vi "CODMn手动控制框.vi"(8 "Error in":errorcluster) -> ()   [LabVIEW 2016, in "斯坦道CODMn.lvlib"]
uses:
  <vilib>/Plasmionique/MB Master/MB Master.lvlib
panel:
  out "退出 2":bool
  in  "采水泵排":bool
  in  "采水泵进":bool
  in  "草酸钠":bool
  in  "高锰酸钾":bool
  in  "高锰酸钾滴定（10uL每滴）":bool
  in  "草酸钠泵排":bool
  in  "草酸钠泵进":bool
  in  "草酸钠泵复位":bool
  in  "高锰酸钾泵排":bool
  in  "高锰酸钾泵进":bool
  in  "高锰酸钾泵复位":bool
  in  "风扇":bool
  in  "排液":bool
  in  "搅拌":bool
  in  "加热":bool
  in  "硫酸":bool
  in  "加标回收样":bool
  in  "零点核查样":bool
  in  "标液":bool
  in  "纯水":bool
  in  "退出":bool
  in  "水样":bool
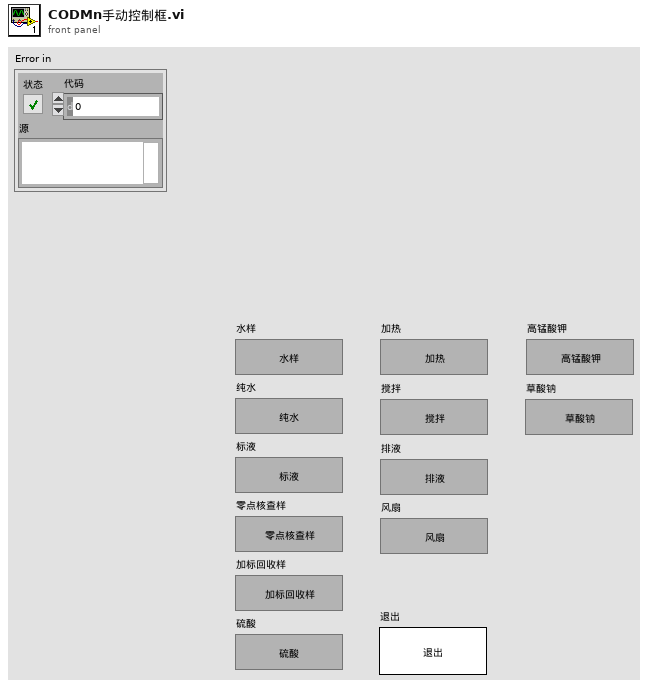
[diagram p1: front panel]
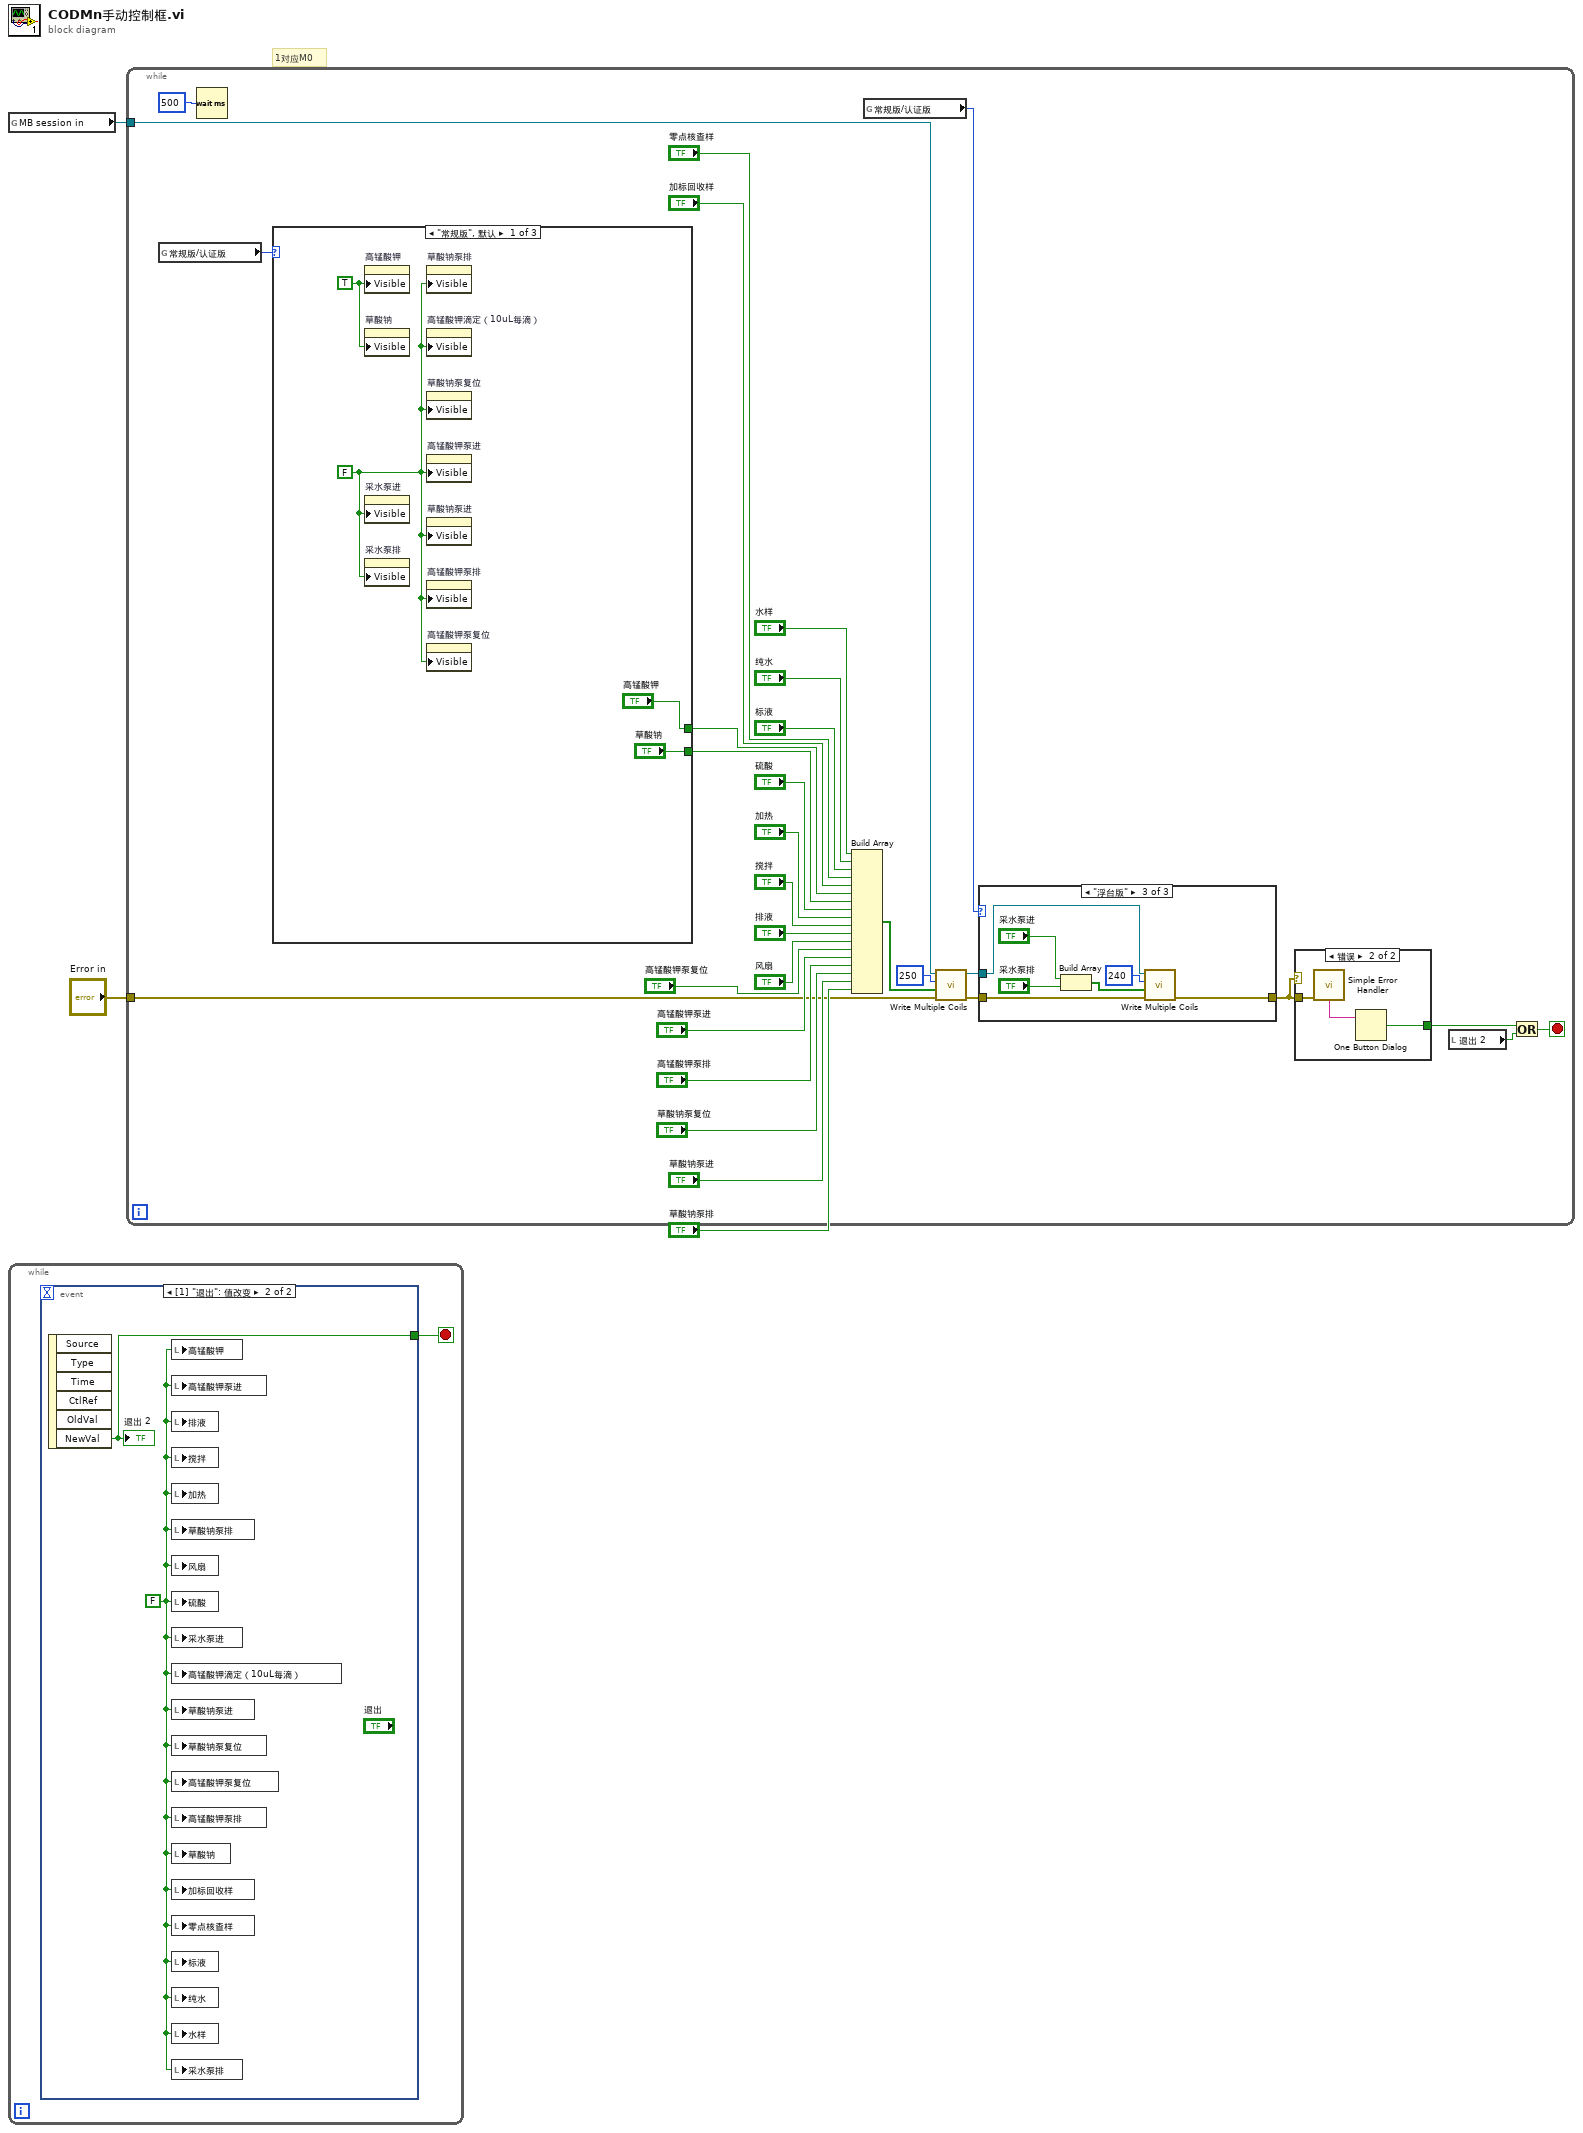
[diagram p0: block diagram]
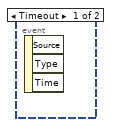
[diagram p2: hidden frame]
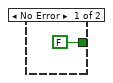
[diagram p3: hidden frame]
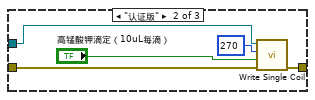
[diagram p5: hidden frame]
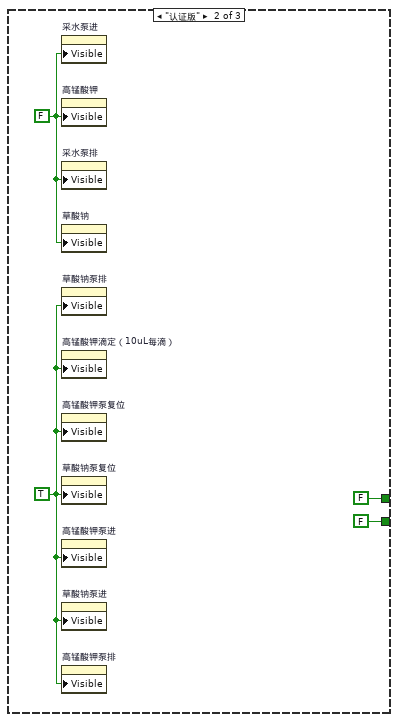
[diagram p6: hidden frame]
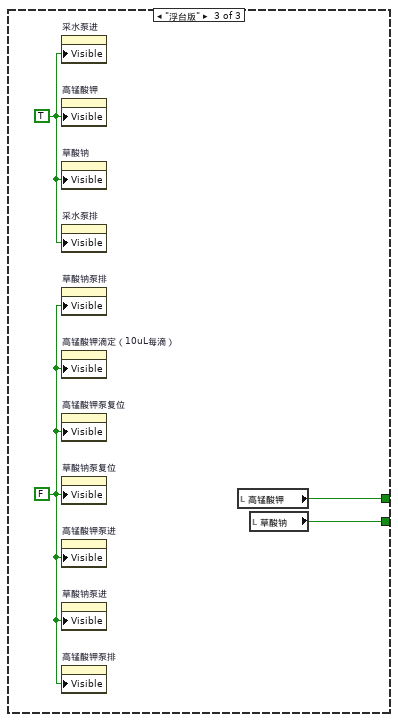
[diagram p7: hidden frame]
diagram:
  # "1对应M0"
  n1 = global read "COD浓度全局变量.vi" "MB session in"() -> (w1:refnum<class "MB_Master.lvclass">)
  n2 = while {
    stop <- w3 stop-if-true
    n3 = event shown="[1] \"退出\": 值改变" {
      selector: _ -> [_ _]
      dyn-events: _ -> [_ _]
      timeout: _ -> [_ _]
      tunnel: [_ w5] -> w3
      event Timeout {
        n4 = event-data() -> ()  [unwired: 1 in, 3 out]
      }
      event "退出": Value Change {
        w4 = FALSE ("草酸钠")
        n5 = event-data() -> ("NewVal"=w5:bool)  [unwired: 1 in, 5 out]
        "退出 2" <- w5
        n6 = local write "高锰酸钾"(w4) -> ()
        n7 = local write "高锰酸钾泵进"(w4) -> ()
        n8 = local write "排液"(w4) -> ()
        n9 = local write "搅拌"(w4) -> ()
        n10 = local write "加热"(w4) -> ()
        n11 = local write "草酸钠泵排"(w4) -> ()
        n12 = local write "风扇"(w4) -> ()
        n13 = local write "硫酸"(w4) -> ()
        n14 = local write "采水泵进"(w4) -> ()
        n15 = local write "高锰酸钾滴定（10uL每滴）"(w4) -> ()
        n16 = local write "草酸钠泵进"(w4) -> ()
        n17 = local write "草酸钠泵复位"(w4) -> ()
        n18 = local write "高锰酸钾泵复位"(w4) -> ()
        n19 = local write "高锰酸钾泵排"(w4) -> ()
        n20 = local write "草酸钠"(w4) -> ()
        n21 = local write "加标回收样"(w4) -> ()
        n22 = local write "零点核查样"(w4) -> ()
        n23 = local write "标液"(w4) -> ()
        n24 = local write "纯水"(w4) -> ()
        n25 = local write "水样"(w4) -> ()
        n26 = local write "采水泵排"(w4) -> ()
      }
    }
  }
  n27 = while {
    tunnel: "Error in" -> [w17]
    tunnel: w1 -> [w12]
    stop <- w9 stop-if-true
    n28 = global read "CODMn断电保存全局变量.vi" "常规版/认证版"() -> (w8:enum16{"常规版", "认证版", "浮台版"})
    n29 = Wait (ms)(milliseconds to wait=u32 500 ("等待时间（毫秒）")) -> ()  [unwired: 1 out]
    n30 = case shown="\"常规版\", 默认" w8 {
      tunnel: ["高锰酸钾" FALSE ("元素") w64] -> w14
      tunnel: ["草酸钠" FALSE ("元素") w63] -> w13
      frame "常规版", Default {
        w54 = FALSE ("可见")
        w57 = TRUE ("可见")
        n31 = property on="高锰酸钾" class="Bool (严格)"("Visible"=w57) -> ()  [unwired: 2 in, 2 out]
        n32 = property on="草酸钠" class="Bool (严格)"("Visible"=w57) -> ()  [unwired: 2 in, 2 out]
        n33 = property on="采水泵进" class="Bool (严格)"("Visible"=w54) -> ()  [unwired: 2 in, 2 out]
        n34 = property on="采水泵排" class="Bool (严格)"("Visible"=w54) -> ()  [unwired: 2 in, 2 out]
        n35 = property on="草酸钠泵排" class="Bool (严格)"("Visible"=w54) -> ()  [unwired: 2 in, 2 out]
        n36 = property on="高锰酸钾滴定（10uL每滴）" class="Bool (严格)"("Visible"=w54) -> ()  [unwired: 2 in, 2 out]
        n37 = property on="草酸钠泵复位" class="Bool (严格)"("Visible"=w54) -> ()  [unwired: 2 in, 2 out]
        n38 = property on="高锰酸钾泵进" class="Bool (严格)"("Visible"=w54) -> ()  [unwired: 2 in, 2 out]
        n39 = property on="草酸钠泵进" class="Bool (严格)"("Visible"=w54) -> ()  [unwired: 2 in, 2 out]
        n40 = property on="高锰酸钾泵排" class="Bool (严格)"("Visible"=w54) -> ()  [unwired: 2 in, 2 out]
        n41 = property on="高锰酸钾泵复位" class="Bool (严格)"("Visible"=w54) -> ()  [unwired: 2 in, 2 out]
      }
      frame "认证版" {
        w61 = TRUE ("可见")
        w58 = FALSE ("可见")
        n42 = property on="采水泵进" class="Bool (严格)"("Visible"=w58) -> ()  [unwired: 2 in, 2 out]
        n43 = property on="高锰酸钾" class="Bool (严格)"("Visible"=w58) -> ()  [unwired: 2 in, 2 out]
        n44 = property on="采水泵排" class="Bool (严格)"("Visible"=w58) -> ()  [unwired: 2 in, 2 out]
        n45 = property on="草酸钠" class="Bool (严格)"("Visible"=w58) -> ()  [unwired: 2 in, 2 out]
        n46 = property on="草酸钠泵排" class="Bool (严格)"("Visible"=w61) -> ()  [unwired: 2 in, 2 out]
        n47 = property on="高锰酸钾滴定（10uL每滴）" class="Bool (严格)"("Visible"=w61) -> ()  [unwired: 2 in, 2 out]
        n48 = property on="高锰酸钾泵复位" class="Bool (严格)"("Visible"=w61) -> ()  [unwired: 2 in, 2 out]
        n49 = property on="草酸钠泵复位" class="Bool (严格)"("Visible"=w61) -> ()  [unwired: 2 in, 2 out]
        n50 = property on="高锰酸钾泵进" class="Bool (严格)"("Visible"=w61) -> ()  [unwired: 2 in, 2 out]
        n51 = property on="草酸钠泵进" class="Bool (严格)"("Visible"=w61) -> ()  [unwired: 2 in, 2 out]
        n52 = property on="高锰酸钾泵排" class="Bool (严格)"("Visible"=w61) -> ()  [unwired: 2 in, 2 out]
      }
      frame "浮台版" {
        w65 = FALSE ("可见")
        w62 = TRUE ("可见")
        n53 = property on="采水泵进" class="Bool (严格)"("Visible"=w62) -> ()  [unwired: 2 in, 2 out]
        n54 = property on="高锰酸钾" class="Bool (严格)"("Visible"=w62) -> ()  [unwired: 2 in, 2 out]
        n55 = property on="草酸钠" class="Bool (严格)"("Visible"=w62) -> ()  [unwired: 2 in, 2 out]
        n56 = property on="采水泵排" class="Bool (严格)"("Visible"=w62) -> ()  [unwired: 2 in, 2 out]
        n57 = property on="草酸钠泵排" class="Bool (严格)"("Visible"=w65) -> ()  [unwired: 2 in, 2 out]
        n58 = property on="高锰酸钾滴定（10uL每滴）" class="Bool (严格)"("Visible"=w65) -> ()  [unwired: 2 in, 2 out]
        n59 = property on="高锰酸钾泵复位" class="Bool (严格)"("Visible"=w65) -> ()  [unwired: 2 in, 2 out]
        n60 = property on="草酸钠泵复位" class="Bool (严格)"("Visible"=w65) -> ()  [unwired: 2 in, 2 out]
        n61 = property on="高锰酸钾泵进" class="Bool (严格)"("Visible"=w65) -> ()  [unwired: 2 in, 2 out]
        n62 = property on="草酸钠泵进" class="Bool (严格)"("Visible"=w65) -> ()  [unwired: 2 in, 2 out]
        n63 = property on="高锰酸钾泵排" class="Bool (严格)"("Visible"=w65) -> ()  [unwired: 2 in, 2 out]
        n64 = local read "高锰酸钾"() -> (w64:bool)
        n65 = local read "草酸钠"() -> (w63:bool)
      }
    }
    n66 = Build Array("水样", "纯水", "标液", "零点核查样", "加标回收样", w14, w13, "硫酸", "加热", "搅拌", "排液", "风扇", "高锰酸钾泵复位", "高锰酸钾泵进", "高锰酸钾泵排", "草酸钠泵复位", "草酸钠泵进", "草酸钠泵排") -> (w34:bool[])
    n67 = global read "CODMn断电保存全局变量.vi" "常规版/认证版"() -> (w7:enum16{"常规版", "认证版", "浮台版"})
    n68 = call <vilib>:"Write Multiple Coils.vi"("error in (no error)"=w17, "values"=w34, "starting address"=u16 250, "MB session in"=w12) -> ("error out"=w15:errorcluster, "MB session out"=w16:refnum<class "MB_Master.lvclass">)  [unwired: 6 in]
    n69 = case shown="\"浮台版\"" w7 {
      tunnel: w16 -> [_ w46 w53]
      tunnel: w15 -> [w41 w45 w52]
      tunnel: [w41 w42 w47] -> w11
      frame "常规版", Default {
      }
      frame "认证版" {
        n70 = call <vilib>:"Write Single Coil.vi"("error in (no error)"=w45, "value"="高锰酸钾滴定（10uL每滴）", "address"=u16 270 ("starting address"), "MB session in"=w46) -> ("error out"=w42:errorcluster)  [unwired: 6 in, 1 out]
      }
      frame "浮台版" {
        n71 = Build Array("采水泵进", "采水泵排") -> (w48:bool[])
        n72 = call <vilib>:"Write Multiple Coils.vi"("error in (no error)"=w52, "values"=w48, "starting address"=u16 240, "MB session in"=w53) -> ("error out"=w47:errorcluster)  [unwired: 6 in, 1 out]
      }
    }
    n73 = case shown="错误" w11 {
      tunnel: w11 -> [_ w40]
      tunnel: [FALSE ("true") w38] -> w10
      frame No Error {
      }
      frame Error {
        n74 = call <vilib>:"Simple Error Handler.vi"("error in (no error)"=w40) -> ("message"=w39:string)  [unwired: 4 in, 4 out]
        n75 = One Button Dialog(message=w39) -> (true=w38:bool)  [unwired: 1 in]
      }
    }
    n76 = local read "退出 2"() -> (w6:bool)
    n77 = Or(x=w10, y=w6) -> (x .or. y?=w9:bool)
  }
